vi "DataCSVFileInfo.vi"(9 "Language":u32, 11 "file path (dialog if empty)":path caption="文件路径 （空时为对话框）") -> (0 "路径输出":path, 1 "FileInfo":string, 2 "文件类型":string)   [LabVIEW 2015]
uses:
  <vilib>/regexp/Match Regular Expression.xnode
panel:
  out "判断":string
  out "末行":string
  out "数据首行":string
  out "行首":string
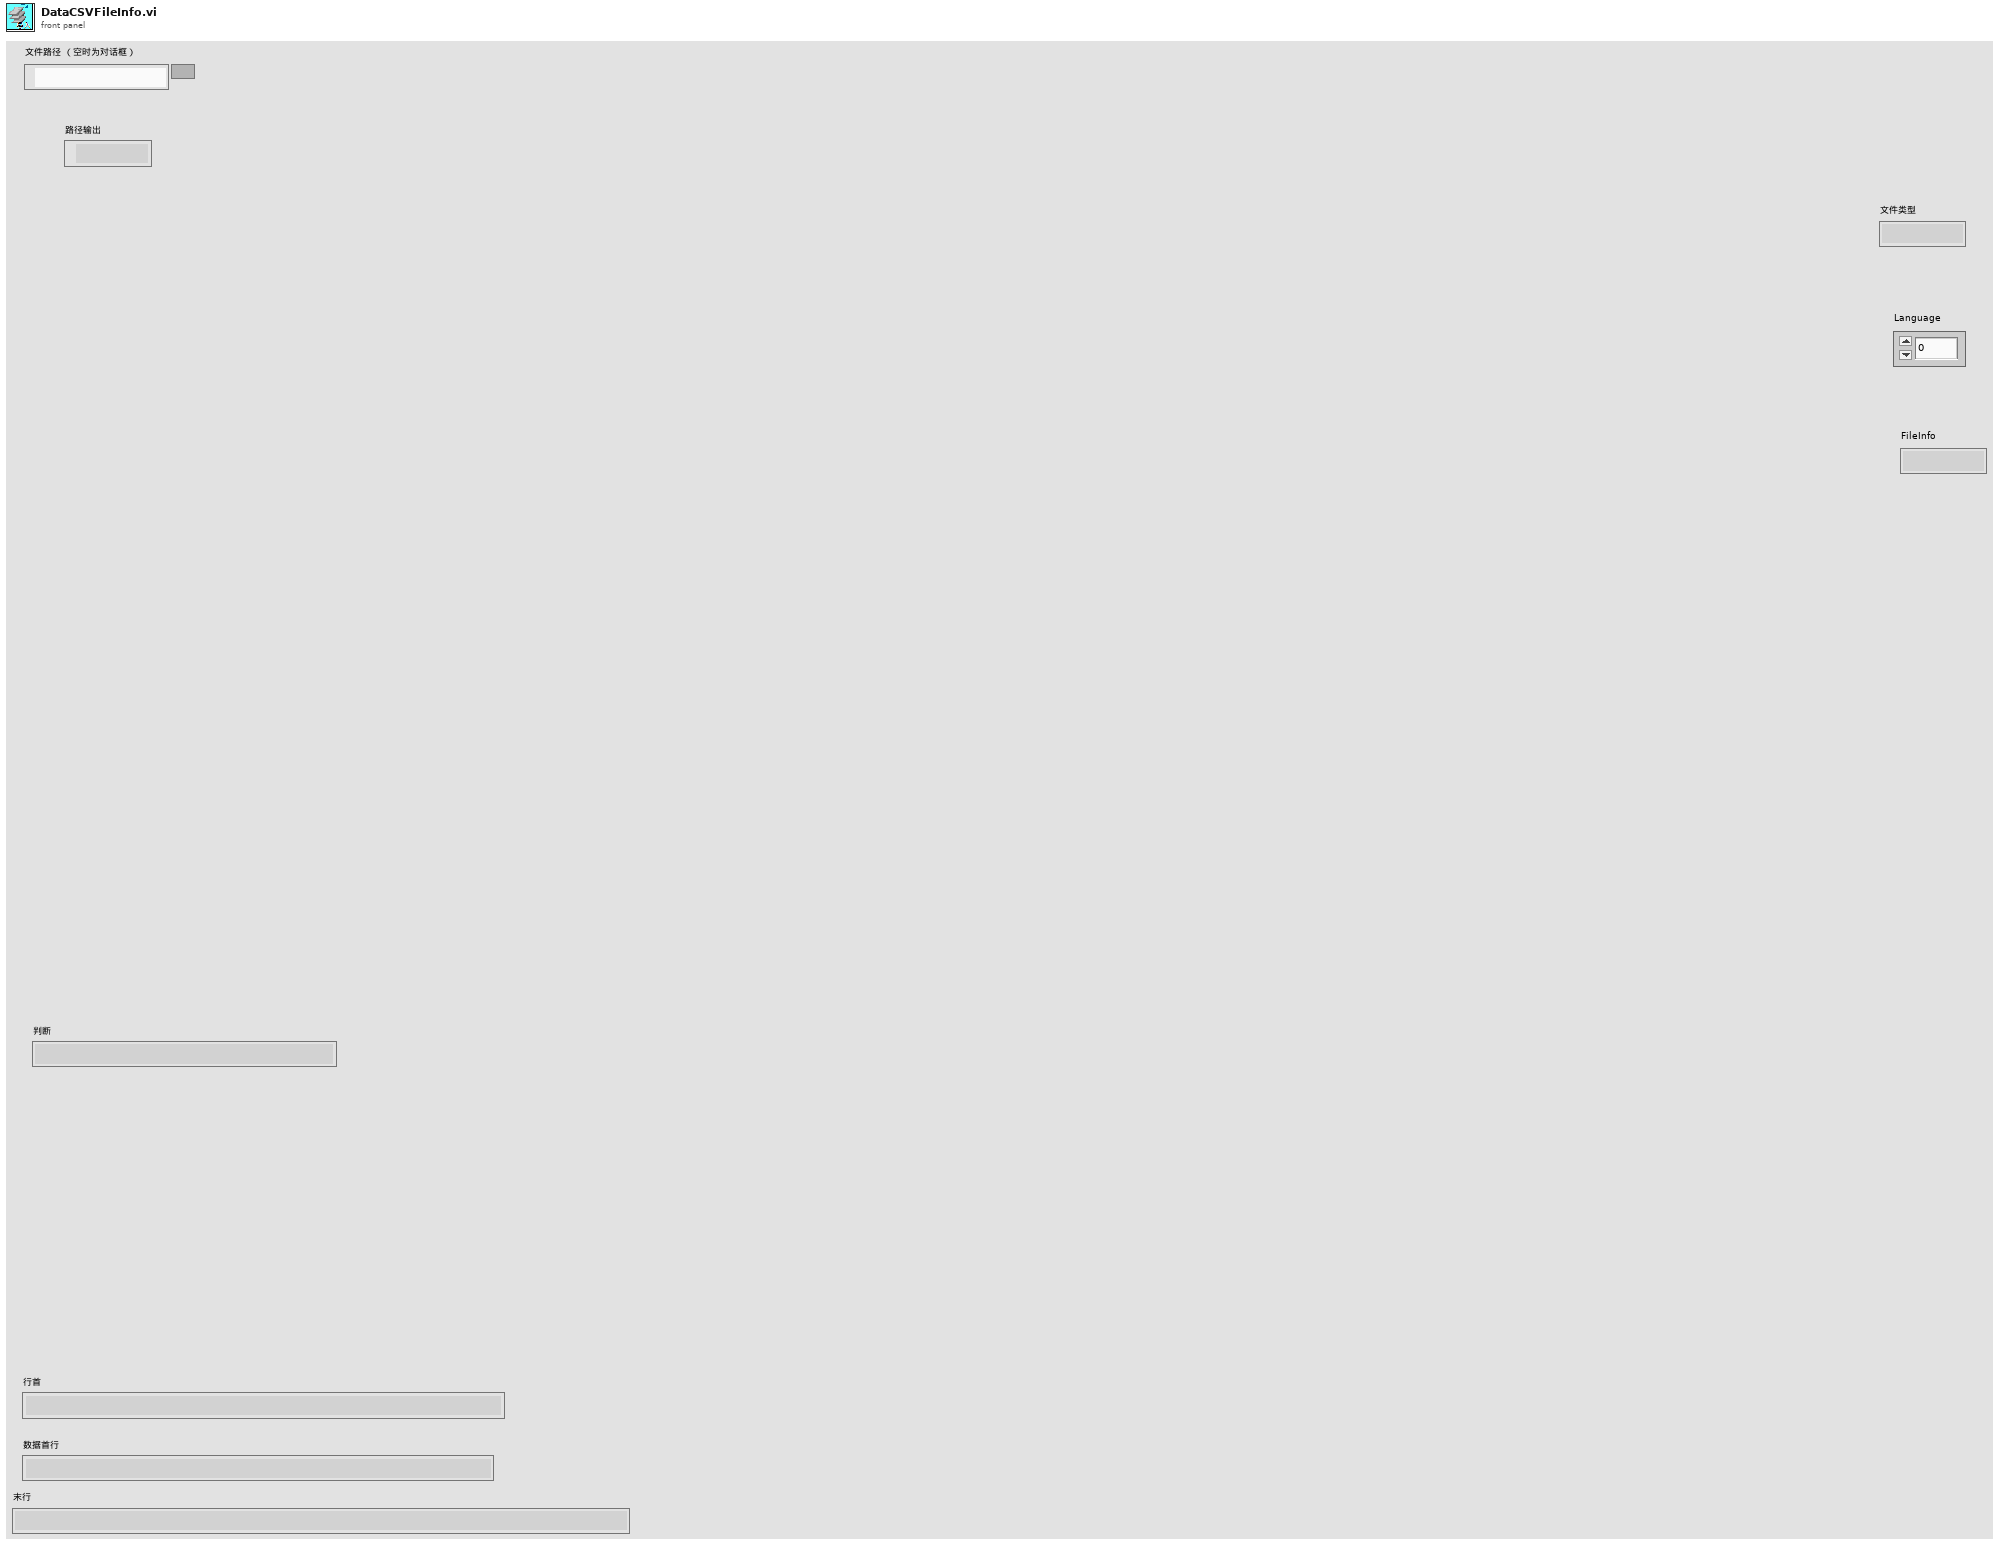
[diagram p1: front panel]
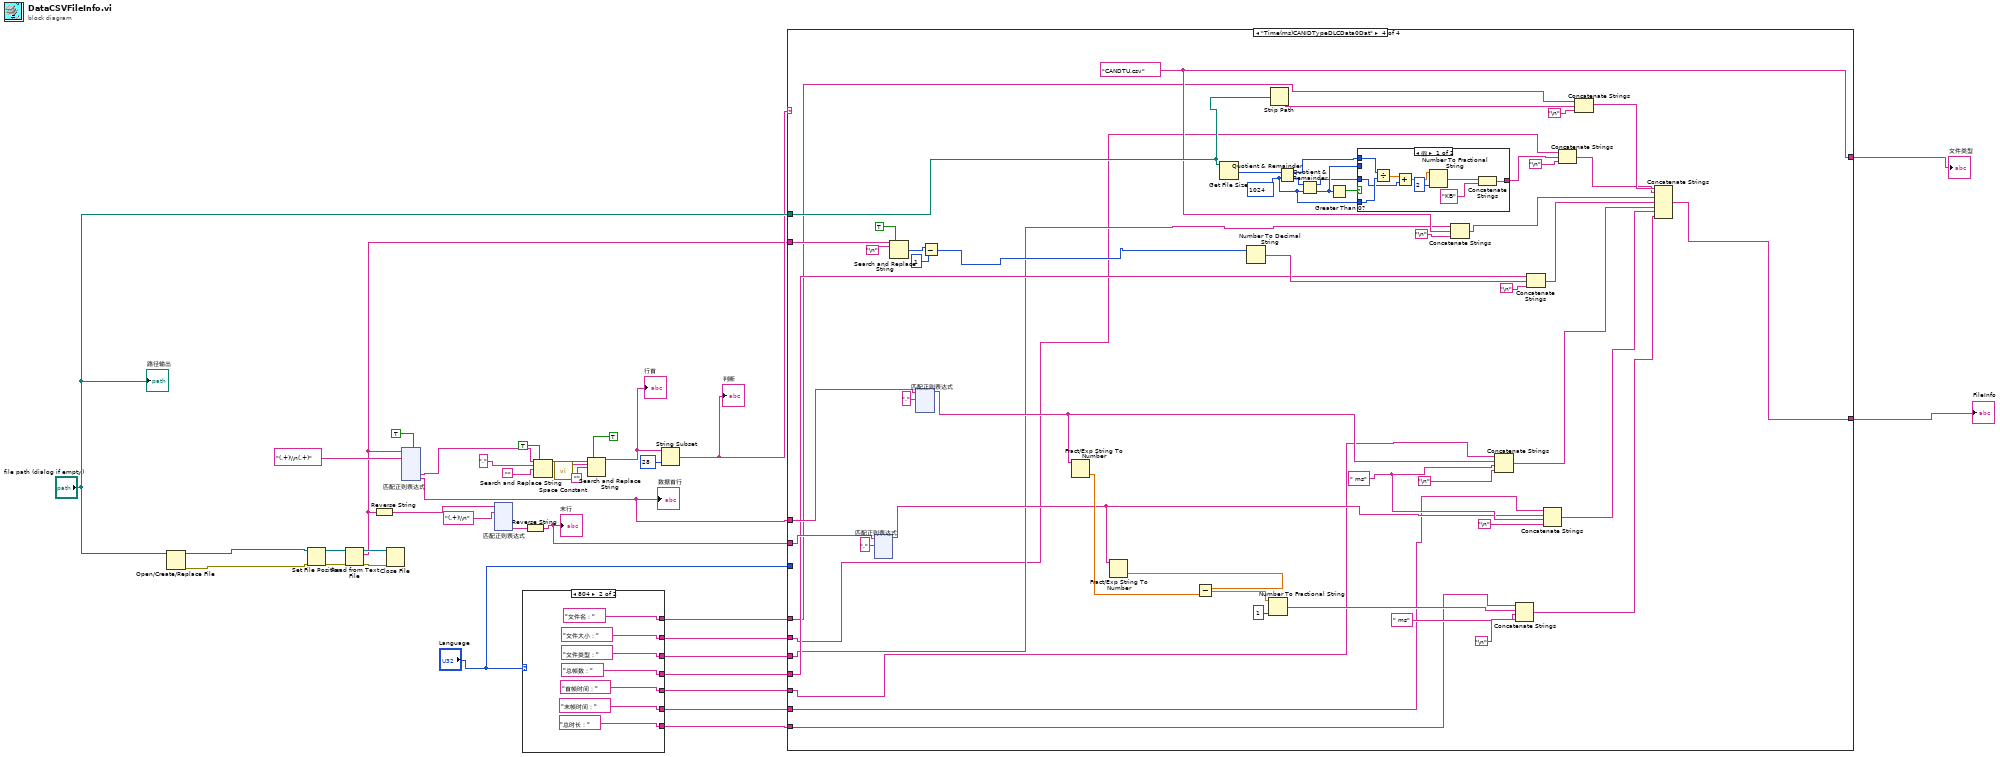
[diagram p0: block diagram]
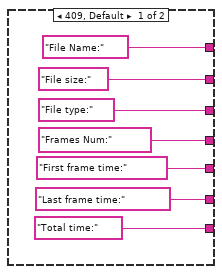
[diagram p2: hidden frame]
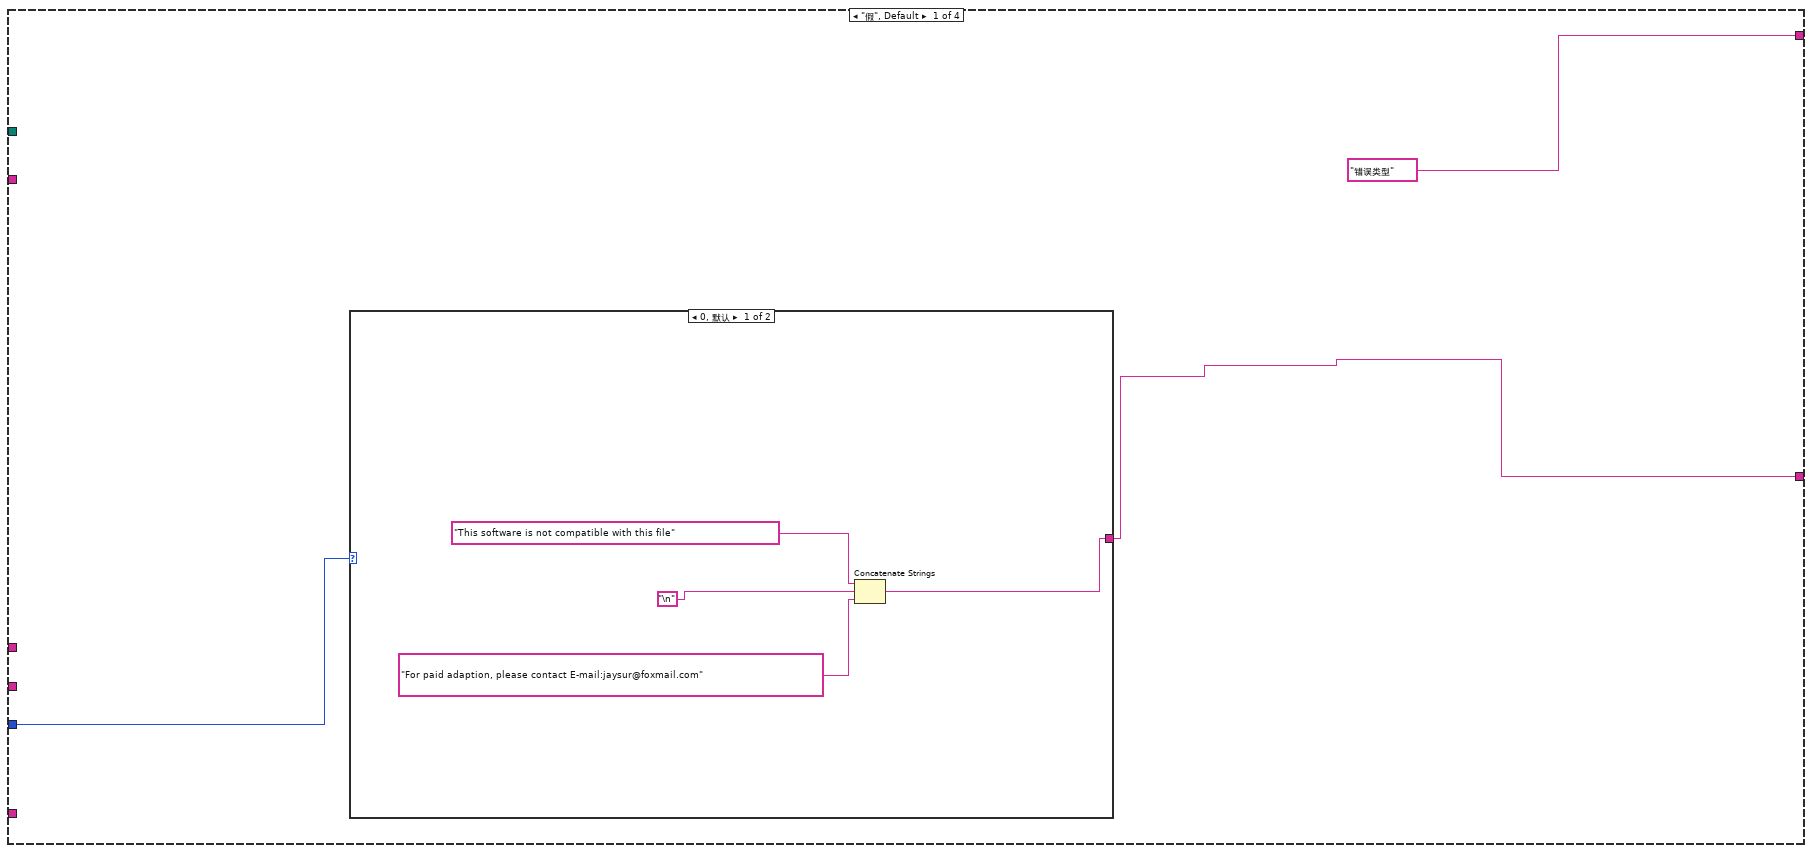
[diagram p3: hidden frame]
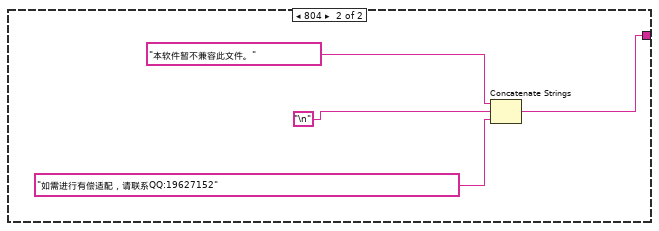
[diagram p4: hidden frame]
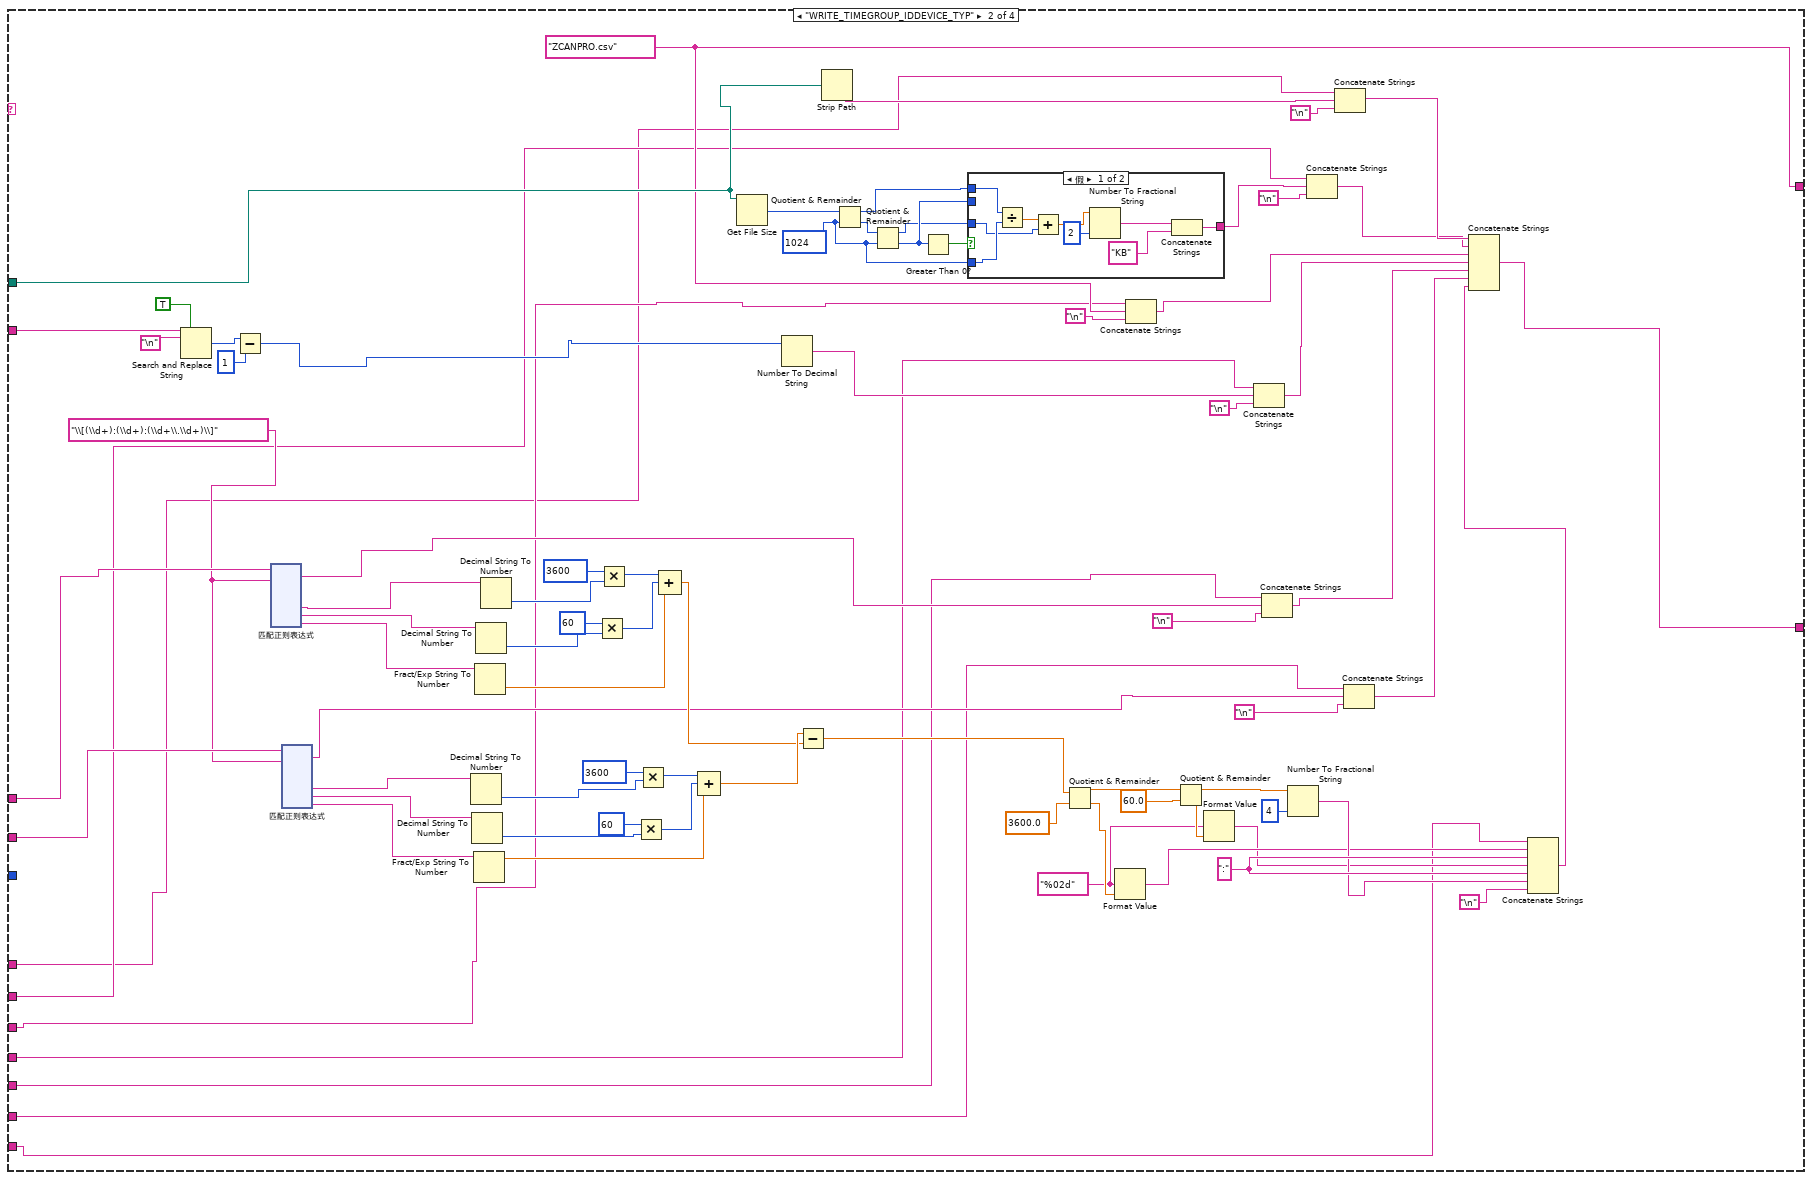
[diagram p5: hidden frame]
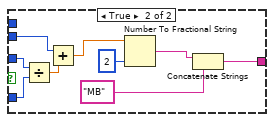
[diagram p6: hidden frame]
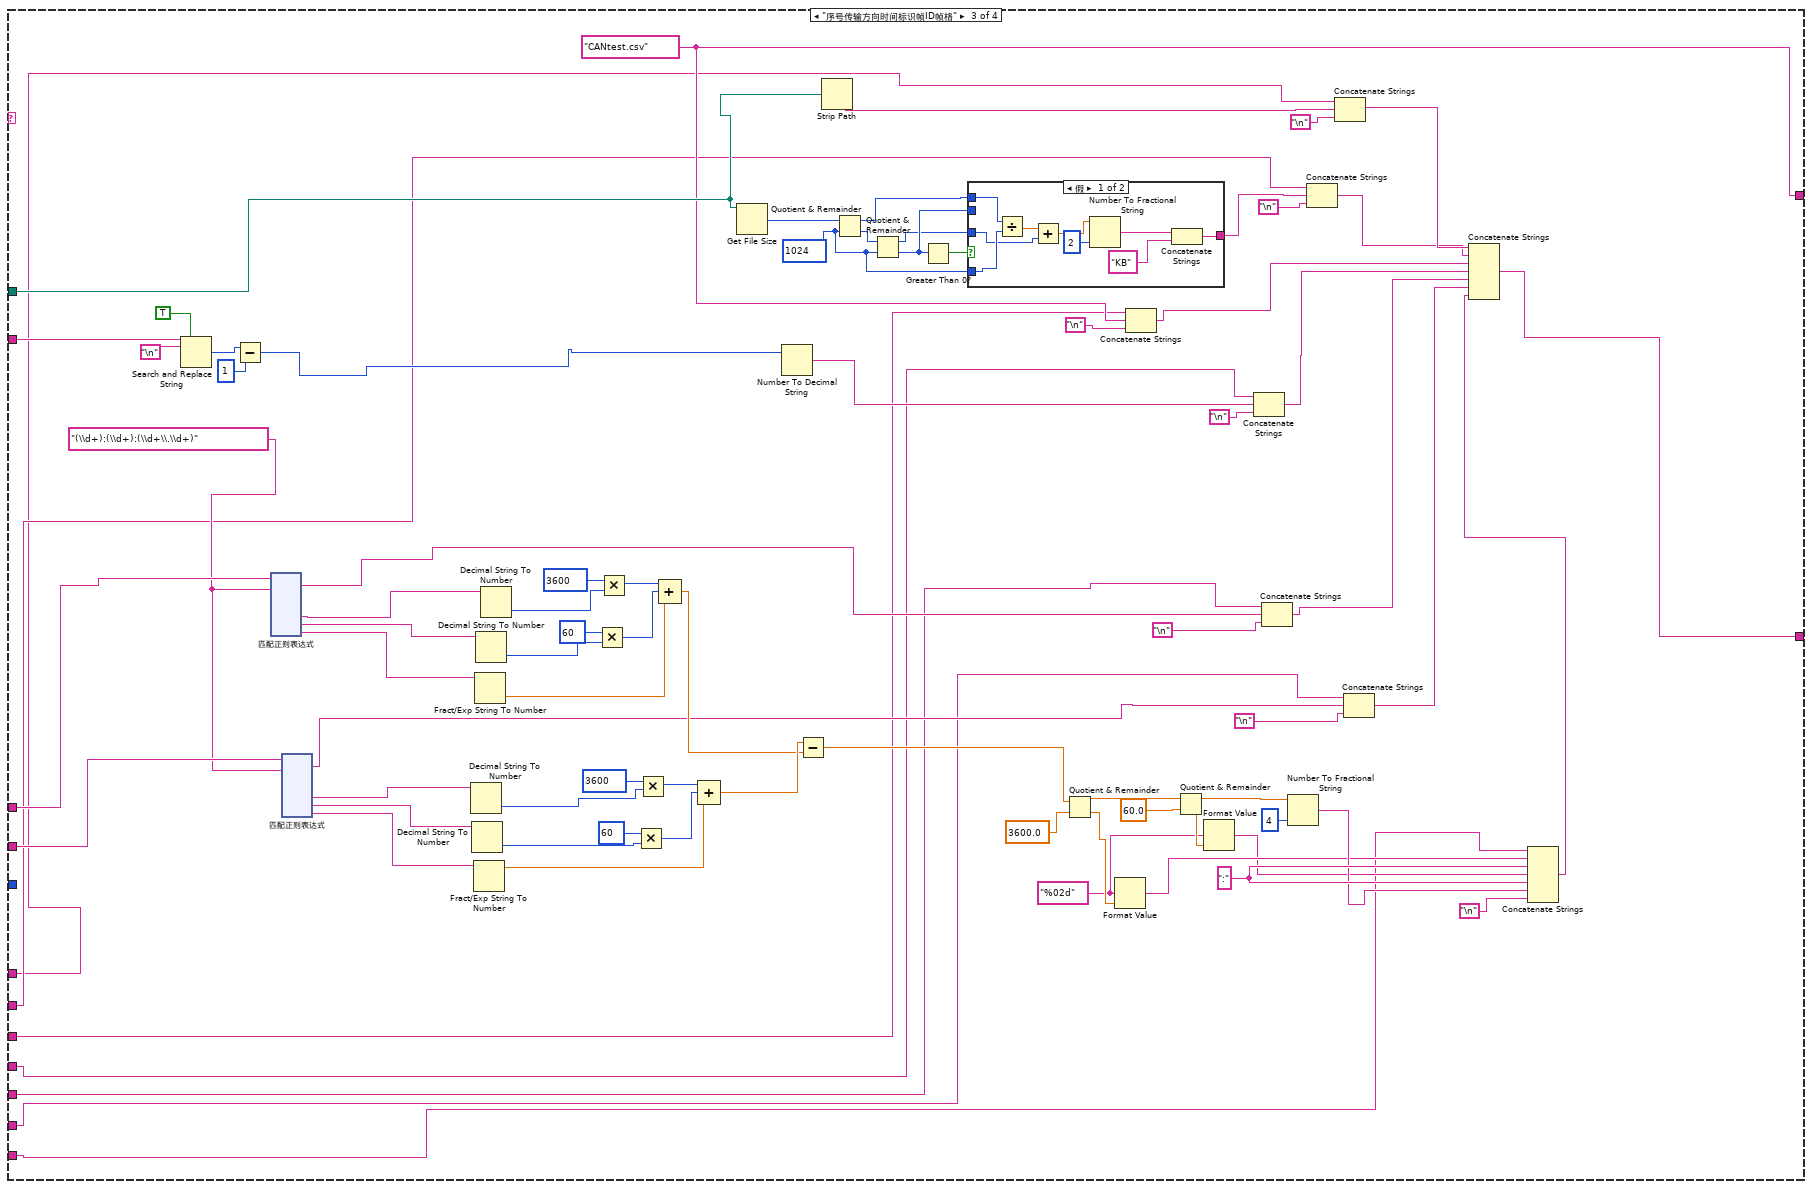
[diagram p7: hidden frame]
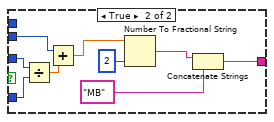
[diagram p8: hidden frame]
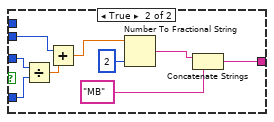
[diagram p9: hidden frame]
diagram:
  n1 = Open/Create/Replace File(file path (use dialog)="file path (dialog if empty)") -> (refnum out=w10:refnum<file>, error out=w9:errorcluster)  [unwired: 5 in, 1 out]
  n2 = Set File Position(refnum=w10, error in=w9) -> (refnum out=w34:refnum<file>, error out=w33:errorcluster)  [unwired: 2 in]
  n3 = Read from Text File(file (use dialog)=w34, error in=w33) -> (refnum out=w18:refnum<file>, text=w11:string, error out=w17:errorcluster)  [unwired: 2 in, 1 out]
  n4 = Reverse String(1:w11) -> (0:w22:string)
  n5 = Close File(refnum=w18, error in=w17) -> ()  [unwired: 2 out]
  n6 = xnode "匹配正则表达式"("输入字符串"=w11, "正则表达式"="(.+)\\n(.+)", "多行？(F)"=TRUE) -> ("子匹配 1"=w29:string, "子匹配 2"=w13:string)  [unwired: 3 in, 5 out]
  "数据首行" <- w13
  n7 = xnode "匹配正则表达式"("输入字符串"=w22, "正则表达式"="(.+)\\n") -> ("子匹配 1"=w21:string)  [unwired: 4 in, 5 out]
  n8 = case shown="804" "Language" {
    tunnel: ["Total time:" "总时长："] -> w2
    tunnel: ["Last frame time:" "末帧时间："] -> w3
    tunnel: ["First frame time:" "首帧时间："] -> w4
    tunnel: ["Frames Num:" "总帧数："] -> w5
    tunnel: ["File type:" "文件类型："] -> w6
    tunnel: ["File size:" "文件大小："] -> w7
    tunnel: ["File Name:" "文件名："] -> w8
    frame 409, Default {
    }
    frame 804 {
    }
  }
  n9 = Reverse String(1:w21) -> (0:w14:string)
  "末行" <- w14
  n10 = Search and Replace String(replace all?=TRUE ("替换全部？(F)"), input string=w29, search string=",", replace string="") -> (result string=w27:string)  [unwired: 4 in, 3 out]
  n11 = call <vilib>:"Space Constant.vi"() -> ("String"=w26:string)
  n12 = Search and Replace String(replace all?=TRUE ("替换全部？(F)"), input string=w27, search string=w26, replace string="") -> (result string=w20:string)  [unwired: 4 in, 3 out]
  "行首" <- w20
  n13 = String Subset(string=w20, length (rest)=28 ("长度（剩余）")) -> (substring=w12:string)  [unwired: 1 in]
  "判断" <- w12
  n14 = case shown="\"Time(ms)CANIDTypeDLCData0Dat\"" w12 {
    tunnel: ["错误类型" w65 w399 w733] -> w36
    tunnel: [w52 w108 w442 w764] -> w35
    tunnel: "file path (dialog if empty)" -> [_ w104 w438 w763]
    tunnel: w14 -> [_ w75 w409 w741]
    tunnel: w13 -> [_ w74 w408 w742]
    tunnel: w11 -> [_ w99 w433 w758]
    tunnel: w8 -> [_ w62 w396 w730]
    tunnel: w7 -> [_ w63 w397 w731]
    tunnel: w6 -> [_ w64 w398 w732]
    tunnel: w5 -> [_ w66 w400 w734]
    tunnel: w4 -> [_ w67 w401 w735]
    tunnel: w3 -> [_ w68 w402 w736]
    tunnel: w2 -> [_ w69 w403 w737]
    tunnel: "Language" -> [w51 _ _ _]
    frame "假", Default {
      n15 = case shown="0, 默认" w51 {
        tunnel: [w54 w58] -> w52
        frame 0, Default {
          n16 = Concatenate Strings("This software is not compatible with this file", "\n", "For paid adaption, please contact E-mail:jaysur@foxmail.com") -> (w54:string)
        }
        frame 804 {
          n17 = Concatenate Strings("本软件暂不兼容此文件。", "\n", "如需进行有偿适配，请联系QQ:19627152") -> (w58:string)
        }
      }
    }
    frame "WRITE_TIMEGROUP_IDDEVICE_TYP" {
      w70 = "\\[(\\d+):(\\d+):(\\d+\\.\\d+)\\]"
      w113 = i64 1024 ("y")
      w130 = "%02d" ("格式字符串")
      w136 = ":"
      w65 = "ZCANPRO.csv"
      n18 = Search and Replace String(replace all?=TRUE ("替换全部？(F)"), input string=w99, search string="\n") -> (number of replacements=w101:i32)  [unwired: 5 in, 3 out]
      n19 = Subtract(x=w101, y=1) -> (x-y=w98:i32)
      n20 = xnode "匹配正则表达式"("输入字符串"=w74, "正则表达式"=w70) -> ("所有匹配"=w71:string, "子匹配 1"=w97:string, "子匹配 2"=w96:string, "子匹配 3"=w95:string)  [unwired: 4 in, 4 out]
      n21 = xnode "匹配正则表达式"("输入字符串"=w75, "正则表达式"=w70) -> ("所有匹配"=w73:string, "子匹配 1"=w94:string, "子匹配 2"=w93:string, "子匹配 3"=w92:string)  [unwired: 4 in, 4 out]
      n22 = Decimal String To Number(string=w94) -> (number=w80:i32)  [unwired: 2 in, 1 out]
      n23 = Decimal String To Number(string=w93) -> (number=w79:i32)  [unwired: 2 in, 1 out]
      n24 = Fract/Exp String To Number(string=w92) -> (number=w78:dbl)  [unwired: 3 in, 1 out]
      n25 = Fract/Exp String To Number(string=w95) -> (number=w85:dbl)  [unwired: 3 in, 1 out]
      n26 = Decimal String To Number(string=w96) -> (number=w91:i32)  [unwired: 2 in, 1 out]
      n27 = Decimal String To Number(string=w97) -> (number=w89:i32)  [unwired: 2 in, 1 out]
      n28 = Multiply(x=60, y=w91) -> (x*y=w86:i32)
      n29 = Multiply(x=3600, y=w89) -> (x*y=w87:i32)
      n30 = Multiply(x=60, y=w79) -> (x*y=w81:i32)
      n31 = Multiply(x=3600, y=w80) -> (x*y=w82:i32)
      n32 = Compound Arithmetic op=ADD(w87, w86, w85) -> (w76:dbl)
      n33 = Compound Arithmetic op=ADD(w82, w81, w78) -> (w77:dbl)
      n34 = Get File Size(file=w104) -> (size (in bytes)=w116:i64)  [unwired: 1 in, 2 out]
      n35 = Number To Decimal String(number=w98) -> (decimal integer string=w119:string)  [unwired: 1 in]
      n36 = Subtract(x=w77, y=w76) -> (x-y=w72:dbl)
      n37 = Strip Path(path=w104) -> (name=w126:string)  [unwired: 1 out]
      n38 = Quotient & Remainder(x=w116, y=w113) -> (x-y*floor(x/y)=w109:i64, floor(x/y)=w115:i64)
      n39 = Quotient & Remainder(x=w115, y=w113) -> (x-y*floor(x/y)=w111:i64, floor(x/y)=w112:i64)
      n40 = Greater Than 0?(x=w112) -> (x > 0?=w114:bool)
      n41 = case shown="假" w114 {
        tunnel: w113 -> [w383 w393]
        tunnel: w112 -> [_ w391]
        tunnel: w111 -> [w381 w394]
        tunnel: [w386 w389] -> w110
        tunnel: w109 -> [w384 _]
        frame False {
          n42 = Divide(x=w384, y=w383) -> (x/y=w382:dbl)
          n43 = Add(x=w382, y=w381) -> (x+y=w380:dbl)
          n44 = Number To Fractional String(number=w380, precision (6)=i16 2 ("精度(6)")) -> (F-format string=w378:string)  [unwired: 2 in]
          n45 = Concatenate Strings(w378, "KB" ("字符串")) -> (w386:string)
        }
        frame True {
          n46 = Divide(x=w394, y=w393) -> (x/y=w392:dbl)
          n47 = Add(x=w391, y=w392) -> (x+y=w390:dbl)
          n48 = Number To Fractional String(number=w390, precision (6)=i16 2 ("精度(6)")) -> (F-format string=w388:string)  [unwired: 2 in]
          n49 = Concatenate Strings(w388, "MB") -> (w389:string)
        }
      }
      n50 = Quotient & Remainder(x=w72, y=3600.0) -> (x-y*floor(x/y)=w140:dbl, floor(x/y)=w133:dbl)
      n51 = Format Value(format string=w130, value (0)=w133) -> (output string=w134:string)  [unwired: 1 in]
      n52 = Concatenate Strings(w64, w65, "\n") -> (w123:string)
      n53 = Quotient & Remainder(x=w140, y=60.0) -> (x-y*floor(x/y)=w138:dbl, floor(x/y)=w132:dbl)
      n54 = Format Value(format string=w130, value (0)=w132) -> (output string=w131:string)  [unwired: 1 in]
      n55 = Concatenate Strings(w66, w119, "\n") -> (w120:string)
      n56 = Concatenate Strings(w67, w71, "\n") -> (w105:string)
      n57 = Number To Fractional String(number=w138, precision (6)=i16 4 ("精度(6)")) -> (F-format string=w135:string)  [unwired: 2 in]
      n58 = Concatenate Strings(w63, w110, "\n") -> (w117:string)
      n59 = Concatenate Strings(w62, w126, "\n") -> (w125:string)
      n60 = Concatenate Strings(w68, w73, "\n") -> (w106:string)
      n61 = Concatenate Strings(w69, w134, w136, w131, w136, w135, "\n") -> (w107:string)
      n62 = Concatenate Strings(w125, w117, w123, w120, w105, w106, w107) -> (w108:string)
    }
    frame "序号传输方向时间标识帧ID帧格" {
      w404 = "(\\d+):(\\d+):(\\d+\\.\\d+)"
      w447 = i64 1024 ("y")
      w464 = "%02d" ("格式字符串")
      w470 = ":"
      w399 = "CANtest.csv"
      n63 = Search and Replace String(replace all?=TRUE ("替换全部？(F)"), input string=w433, search string="\n") -> (number of replacements=w435:i32)  [unwired: 5 in, 3 out]
      n64 = Subtract(x=w435, y=1) -> (x-y=w432:i32)
      n65 = xnode "匹配正则表达式"("输入字符串"=w408, "正则表达式"=w404) -> ("所有匹配"=w405:string, "子匹配 1"=w431:string, "子匹配 2"=w430:string, "子匹配 3"=w429:string)  [unwired: 4 in, 4 out]
      n66 = xnode "匹配正则表达式"("输入字符串"=w409, "正则表达式"=w404) -> ("所有匹配"=w407:string, "子匹配 1"=w428:string, "子匹配 2"=w427:string, "子匹配 3"=w426:string)  [unwired: 4 in, 4 out]
      n67 = Decimal String To Number(string=w428) -> (number=w414:i32)  [unwired: 2 in, 1 out]
      n68 = Decimal String To Number(string=w427) -> (number=w413:i32)  [unwired: 2 in, 1 out]
      n69 = Fract/Exp String To Number(string=w426) -> (number=w412:dbl)  [unwired: 3 in, 1 out]
      n70 = Fract/Exp String To Number(string=w429) -> (number=w419:dbl)  [unwired: 3 in, 1 out]
      n71 = Decimal String To Number(string=w430) -> (number=w425:i32)  [unwired: 2 in, 1 out]
      n72 = Decimal String To Number(string=w431) -> (number=w423:i32)  [unwired: 2 in, 1 out]
      n73 = Multiply(x=60, y=w425) -> (x*y=w420:i32)
      n74 = Multiply(x=3600, y=w423) -> (x*y=w421:i32)
      n75 = Multiply(x=60, y=w413) -> (x*y=w415:i32)
      n76 = Multiply(x=3600, y=w414) -> (x*y=w416:i32)
      n77 = Compound Arithmetic op=ADD(w421, w420, w419) -> (w410:dbl)
      n78 = Compound Arithmetic op=ADD(w416, w415, w412) -> (w411:dbl)
      n79 = Get File Size(file=w438) -> (size (in bytes)=w450:i64)  [unwired: 1 in, 2 out]
      n80 = Number To Decimal String(number=w432) -> (decimal integer string=w453:string)  [unwired: 1 in]
      n81 = Subtract(x=w411, y=w410) -> (x-y=w406:dbl)
      n82 = Strip Path(path=w438) -> (name=w460:string)  [unwired: 1 out]
      n83 = Quotient & Remainder(x=w450, y=w447) -> (x-y*floor(x/y)=w443:i64, floor(x/y)=w449:i64)
      n84 = Quotient & Remainder(x=w449, y=w447) -> (x-y*floor(x/y)=w445:i64, floor(x/y)=w446:i64)
      n85 = Greater Than 0?(x=w446) -> (x > 0?=w448:bool)
      n86 = case shown="假" w448 {
        tunnel: w447 -> [w717 w727]
        tunnel: w446 -> [_ w725]
        tunnel: w445 -> [w715 w728]
        tunnel: [w720 w723] -> w444
        tunnel: w443 -> [w718 _]
        frame False {
          n87 = Divide(x=w718, y=w717) -> (x/y=w716:dbl)
          n88 = Add(x=w716, y=w715) -> (x+y=w714:dbl)
          n89 = Number To Fractional String(number=w714, precision (6)=i16 2 ("精度(6)")) -> (F-format string=w712:string)  [unwired: 2 in]
          n90 = Concatenate Strings(w712, "KB" ("字符串")) -> (w720:string)
        }
        frame True {
          n91 = Divide(x=w728, y=w727) -> (x/y=w726:dbl)
          n92 = Add(x=w725, y=w726) -> (x+y=w724:dbl)
          n93 = Number To Fractional String(number=w724, precision (6)=i16 2 ("精度(6)")) -> (F-format string=w722:string)  [unwired: 2 in]
          n94 = Concatenate Strings(w722, "MB") -> (w723:string)
        }
      }
      n95 = Quotient & Remainder(x=w406, y=3600.0) -> (x-y*floor(x/y)=w474:dbl, floor(x/y)=w467:dbl)
      n96 = Format Value(format string=w464, value (0)=w467) -> (output string=w468:string)  [unwired: 1 in]
      n97 = Concatenate Strings(w398, w399, "\n") -> (w457:string)
      n98 = Quotient & Remainder(x=w474, y=60.0) -> (x-y*floor(x/y)=w472:dbl, floor(x/y)=w466:dbl)
      n99 = Format Value(format string=w464, value (0)=w466) -> (output string=w465:string)  [unwired: 1 in]
      n100 = Concatenate Strings(w400, w453, "\n") -> (w454:string)
      n101 = Concatenate Strings(w401, w405, "\n") -> (w439:string)
      n102 = Number To Fractional String(number=w472, precision (6)=i16 4 ("精度(6)")) -> (F-format string=w469:string)  [unwired: 2 in]
      n103 = Concatenate Strings(w397, w444, "\n") -> (w451:string)
      n104 = Concatenate Strings(w396, w460, "\n") -> (w459:string)
      n105 = Concatenate Strings(w402, w407, "\n") -> (w440:string)
      n106 = Concatenate Strings(w403, w468, w470, w465, w470, w469, "\n") -> (w441:string)
      n107 = Concatenate Strings(w459, w451, w457, w454, w439, w440, w441) -> (w442:string)
    }
    frame "Time(ms)CANIDTypeDLCData0Dat" {
      w751 = " ms"
      w769 = i64 1024 ("y")
      w733 = "CANDTU.csv"
      n108 = xnode "匹配正则表达式"("输入字符串"=w741, "正则表达式"=",") -> ("匹配之前"=w744:string)  [unwired: 4 in, 4 out]
      n109 = Search and Replace String(replace all?=TRUE ("替换全部？(F)"), input string=w758, search string="\n") -> (number of replacements=w760:i32)  [unwired: 5 in, 3 out]
      n110 = xnode "匹配正则表达式"("输入字符串"=w742, "正则表达式"=",") -> ("匹配之前"=w743:string)  [unwired: 4 in, 4 out]
      n111 = Subtract(x=w760, y=1) -> (x-y=w757:i32)
      n112 = Fract/Exp String To Number(string=w743) -> (number=w749:dbl)  [unwired: 3 in, 1 out]
      n113 = Fract/Exp String To Number(string=w744) -> (number=w750:dbl)  [unwired: 3 in, 1 out]
      n114 = Subtract(x=w750, y=w749) -> (x-y=w748:dbl)
      n115 = Get File Size(file=w763) -> (size (in bytes)=w772:i64)  [unwired: 1 in, 2 out]
      n116 = Number To Decimal String(number=w757) -> (decimal integer string=w775:string)  [unwired: 1 in]
      n117 = Number To Fractional String(number=w748, precision (6)=i16 1 ("精度(6)")) -> (F-format string=w746:string)  [unwired: 2 in]
      n118 = Strip Path(path=w763) -> (name=w782:string)  [unwired: 1 out]
      n119 = Quotient & Remainder(x=w772, y=w769) -> (x-y*floor(x/y)=w765:i64, floor(x/y)=w771:i64)
      n120 = Quotient & Remainder(x=w771, y=w769) -> (x-y*floor(x/y)=w767:i64, floor(x/y)=w768:i64)
      n121 = Greater Than 0?(x=w768) -> (x > 0?=w770:bool)
      n122 = case shown="假" w770 {
        tunnel: w769 -> [w1016 w1026]
        tunnel: w768 -> [_ w1024]
        tunnel: w767 -> [w1014 w1027]
        tunnel: [w1019 w1022] -> w766
        tunnel: w765 -> [w1017 _]
        frame False {
          n123 = Divide(x=w1017, y=w1016) -> (x/y=w1015:dbl)
          n124 = Add(x=w1015, y=w1014) -> (x+y=w1013:dbl)
          n125 = Number To Fractional String(number=w1013, precision (6)=i16 2 ("精度(6)")) -> (F-format string=w1011:string)  [unwired: 2 in]
          n126 = Concatenate Strings(w1011, "KB" ("字符串")) -> (w1019:string)
        }
        frame True {
          n127 = Divide(x=w1027, y=w1026) -> (x/y=w1025:dbl)
          n128 = Add(x=w1024, y=w1025) -> (x+y=w1023:dbl)
          n129 = Number To Fractional String(number=w1023, precision (6)=i16 2 ("精度(6)")) -> (F-format string=w1021:string)  [unwired: 2 in]
          n130 = Concatenate Strings(w1021, "MB") -> (w1022:string)
        }
      }
      n131 = Concatenate Strings(w732, w733, "\n") -> (w779:string)
      n132 = Concatenate Strings(w735, w743, w751, "\n") -> (w739:string)
      n133 = Concatenate Strings(w737, w746, " ms", "\n") -> (w740:string)
      n134 = Concatenate Strings(w734, w775, "\n") -> (w776:string)
      n135 = Concatenate Strings(w736, w744, w751, "\n") -> (w738:string)
      n136 = Concatenate Strings(w731, w766, "\n") -> (w773:string)
      n137 = Concatenate Strings(w730, w782, "\n") -> (w781:string)
      n138 = Concatenate Strings(w781, w773, w779, w776, w739, w738, w740) -> (w764:string)
    }
  }
  "FileInfo" <- w35
  "文件类型" <- w36
  "路径输出" <- "file path (dialog if empty)"
